vi "LV Colormap Fresh.vi"(7 "Colormap Name":T1(ring)=enum."vanimo") -> (8 "Colormap":u32[](array[colorbox]))   [LabVIEW 2024]
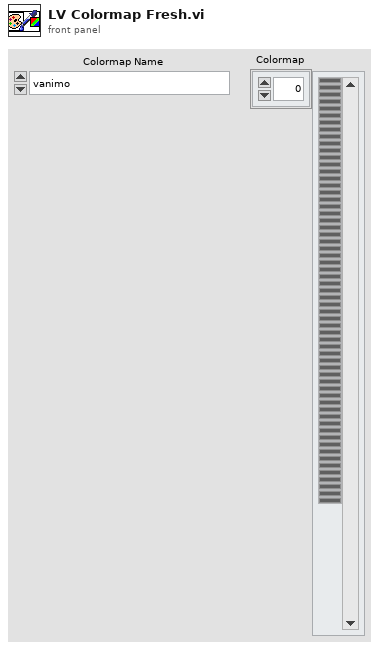
[diagram p1: front panel]
types:
  T1 = enum16{"magma", "inferno", "plasma", "viridis", "cividis", "twilight", "twilight_shifted", "turbo", "berlin", "managua", "vanimo"}
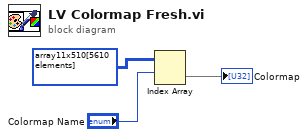
[diagram p0: block diagram]
diagram:
  n1 = Index Array(array=u32[][] array11x510[5610 elements] ("Array 2"), index (row)="Colormap Name") -> (element=→"Colormap":u32[])  [unwired: 1 in]
